vi "OutputData.vi"() -> ()   [LabVIEW 2018]
panel:
  out "数组":dbl[](array[numeric])
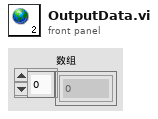
[diagram p1: front panel]
diagram:
